vi "Wait for Acq.vi"(8 "error in (no error)":errorcluster, 11 "Notifier in":refnum<notifier>) -> (0 "error out":errorcluster, 2 "timed out?":bool, 3 "Array":dbl[](array[numeric]))   [LabVIEW 2015]
uses:
  App Data.vi
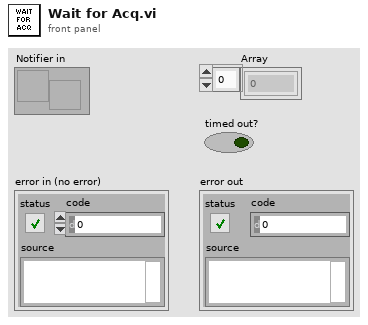
[diagram p1: front panel]
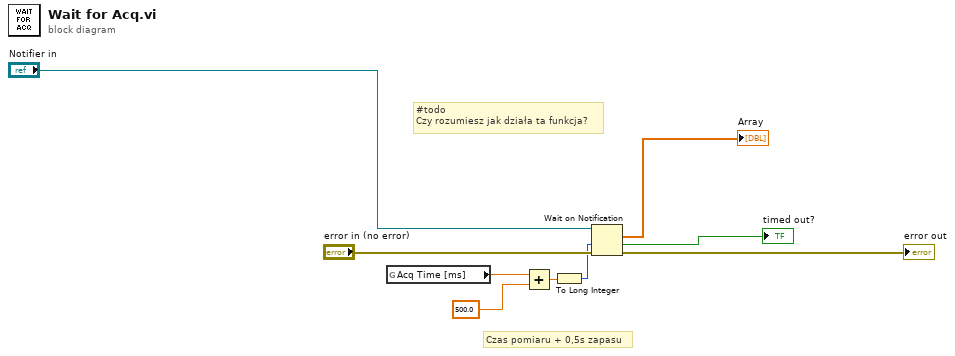
[diagram p0: block diagram]
diagram:
  # "#todo\nCzy rozumiesz jak działa ta funkcja?"
  # "Czas pomiaru + 0,5s zapasu"
  n1 = global read "App Data.vi" "Acq Time [ms]"() -> (w2:dbl)
  n2 = Add(x=w2, y=500.0) -> (x+y=w4:dbl)
  n3 = To Long Integer(number=w4) -> (32bit integer=w5:i32)
  n4 = Wait on Notification(notifier="Notifier in", timeout in ms (-1)=w5, error in (no error)="error in (no error)") -> (notification=→"Array":dbl[], timed out?=→"timed out?":bool, error out=→"error out":errorcluster)  [unwired: 1 in, 1 out]
